vi "Save Image to Disk.vi"(6 "Image Quality":u32=1024, 8 "error in":errorcluster, 10 "Path":path, 11 "BigMAQ in":refnum<class "BigMAQ.lvclass">) -> (0 "error out":errorcluster, 3 "BigMAQ out":refnum<class "BigMAQ.lvclass">)   [LabVIEW 2019, in "BigMAQ.lvclass"]
uses:
  BigMAQ.lvclass
  BigMAQ.lvclass/BigMAQ.ctl
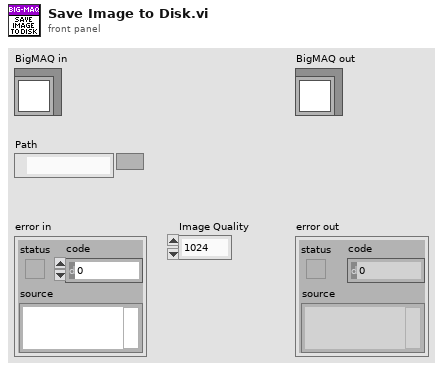
[diagram p1: front panel]
types:
  T1 = typedef "Image Type" = u32
  T2 = typedef "IMAQ Image.ctl" = refnum<image>
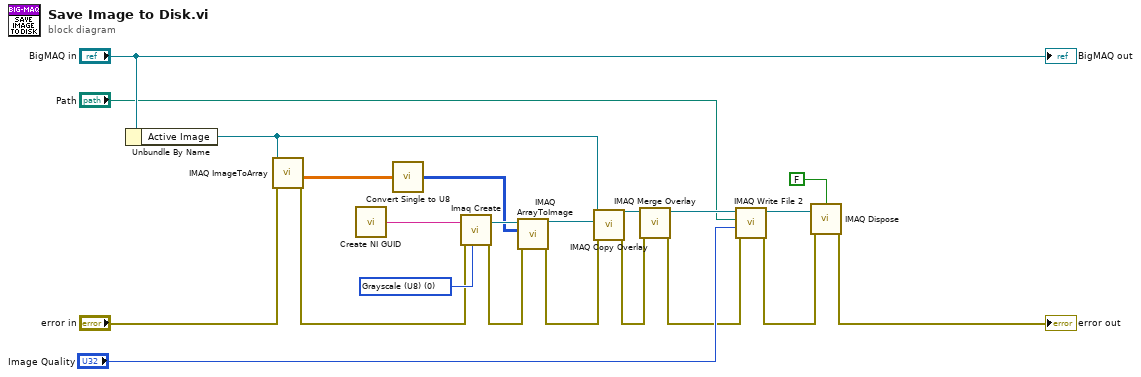
[diagram p0: block diagram]
diagram:
  w18 = T1 0 items=["Grayscale (U8)", "Grayscale (I16)", "Grayscale (SGL)", "Complex (CSG)", "RGB (U32)", "HSL (U32)", "RGB (U64)", "Grayscale (U16)"] ("Image Type")
  n1 = Unbundle By Name("BigMAQ in") -> ("Active Image"=w4:T2)
  n2 = call "IMAQ ImageToArray"("error in (no error)"="error in", "Image"=w4) -> ("Image Pixels (Float)"=w14:sgl[][], "error out"=w2:errorcluster)  [unwired: 2 in, 3 out]
  n3 = call "Create NI GUID.vi"() -> ("NI GUID"=w1:string)
  n4 = call "Convert Single to U8.vi"("Image Pixels (Float)"=w14) -> ("Image Pixels (U8)"=w13:u8[][])
  n5 = call "Imaq Create"("Image Name"=w1, "Image Type"=w18, "error in (no error)"=w2) -> ("New Image"=w16:T2, "error out"=w15:errorcluster)  [unwired: 2 in]
  n6 = call "IMAQ ArrayToImage"("error in (no error)"=w15, "Image Pixels (U8)"=w13, "Image"=w16) -> ("error out"=w10:errorcluster, "Image Out"=w8:T2)  [unwired: 7 in]
  n7 = call "IMAQ Copy Overlay"("error in (no error)"=w10, "Image Dst"=w8, "Image Src"=w4) -> ("error out"=w6:errorcluster, "Image Dst Out"=w9:T2)  [unwired: 7 in]
  n8 = call "IMAQ Merge Overlay"("error in (no error)"=w6, "Image Src"=w9) -> ("error out"=w5:errorcluster, "Image Dst Out"=w7:T2)  [unwired: 8 in]
  n9 = call-poly "IMAQ Write File 2"("error in (no error)"=w5, "Image Quality"="Image Quality", "File Path"="Path", "Image"=w7) -> ("error out"=w17:errorcluster, "Image Out (duplicate)"=w19:T2)  [unwired: 6 in]
  n10 = call "IMAQ Dispose"("All Images? (No)"=FALSE, "Image"=w19, "error in (no error)"=w17) -> ("error out"=→"error out":errorcluster)  [unwired: 3 in]
  "BigMAQ out" <- "BigMAQ in"
